vi "First Step.vi"(8 "error in (no error)":errorcluster, 11 "Varian Continuous.lvclass in":refnum<class "Varian Continuous.lvclass">) -> (0 "error out":errorcluster, 2 "Current Position":dbl, 3 "Varian Continuous.lvclass out":refnum<class "Varian Continuous.lvclass">)   [LabVIEW 2009, in "Varian Continuous.lvclass"]
doc: "(Dynamic) Reset the instrument and prepare to scan. Go to step #0 - the first step. If desired, the scanner may do this in a different way than usual (i.e. by preparing to move a long distance, or reset to home position.)"
uses:
  Varian Continuous.lvclass
  Instruments/Varian Magnet/Varian Magnet.lvclass
  Scanner/Scanner.lvclass
  Instruments/Varian Magnet/Varian Max Field.vi
  Varian Continuous.lvclass/Varian Continuous.ctl
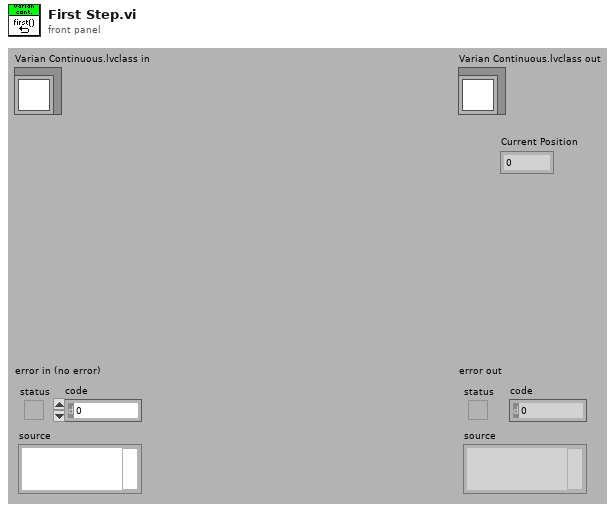
[diagram p1: front panel]
types:
  T1 = typedef "Scanner.lvclass/Range.ctl" = cluster{"xi":dbl, "xf":dbl, "dx":dbl, "Return to...?":bool, "Return to":dbl}
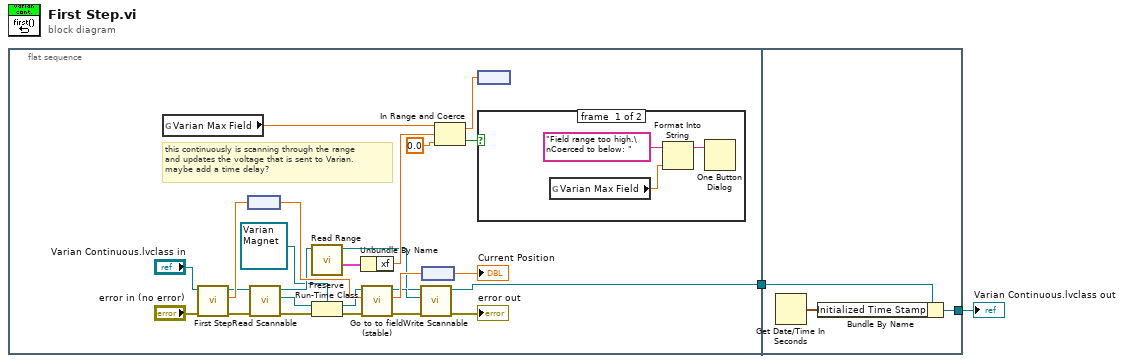
[diagram p0: block diagram]
diagram:
  n1 = flat-sequence {
    tunnel: [w10] -> w2
    tunnel: w2 -> [w32]
    tunnel: [w31] -> w1
    frame #0 {
      # "this continuously is scanning through the range\nand updates the voltage that is sent to Varian.\nmaybe add a time delay?"
      n2 = global read "Varian Max Field.vi" "Varian Max Field"() -> (w20:dbl[unit])
      n3 = call-parent "First Step.vi"("error in (no error)"="error in (no error)", "Scanner.lvclass in"="Varian Continuous.lvclass in") -> ("error out"=w13:errorcluster, "Current Position"=w25:dbl, "Scanner.lvclass out"=w21:refnum<class "Varian Continuous.lvclass">)  [unwired: 7 in]
      n4 = node(w25) -> (w24:dbl[unit])
      n5 = call-dynamic "Read Scannable.vi"("error in (no error)"=w13, "Scanner.lvclass in"=w21) -> ("error out"=w4:errorcluster, "Scannable.lvclass"=w7:refnum<class "Scannable.lvclass">, "Scanner.lvclass out"=w16:refnum<class "Varian Continuous.lvclass">)  [unwired: 7 in]
      n6 = call-dynamic "Read Range.vi"("Scanner.lvclass in"=w16) -> ("Range"=w15:T1, "Scanner.lvclass out"=w11:refnum<class "Varian Continuous.lvclass">)  [unwired: 5 in, 4 out]
      n7 = Preserve Run-Time Class(object in=w7, error in=w4, 2:refnum<class "Varian Magnet.lvclass"> refnum ("Varian Magnet.lvclass")) -> (object out=w5:refnum<class "Varian Magnet.lvclass">, error out=w3:errorcluster)
      n8 = Unbundle By Name(w15) -> ("xf"=w14:dbl)
      n9 = call "Go to to field (stable).vi"("error in"=w3, "Desired field"=w24, "varian in"=w5) -> ("error out"=w8:errorcluster, "Current field"=w22:dbl[unit], "varian out"=w12:refnum<class "Varian Magnet.lvclass">)  [unwired: 5 in, 1 out]
      n10 = call-dynamic "Write Scannable.vi"("error in (no error)"=w8, "Scannable.lvclass"=w12, "Scanner.lvclass in"=w11) -> ("error out"=→"error out":errorcluster, "Scanner.lvclass out"=w10:refnum<class "Varian Continuous.lvclass">)  [unwired: 7 out]
      n11 = node(w22) -> (→"Current Position":dbl)
      n12 = In Range and Coerce(upper limit=w20, x=w14, lower limit=dbl[unit] 0.0) -> (coerced(x)=w18:dbl[unit], In Range?=w17:bool)
      n13 = node(w18) -> ()  [unwired: 1 out]
      n14 = case shown="False" w17 {
        frame #0 {
          n15 = global read "Varian Max Field.vi" "Varian Max Field"() -> (w28:dbl[unit])
          n16 = Format Into String(initial string="Field range too high.\nCoerced to below: " ("message"), w28) -> (resulting string=w30:string)  [unwired: 2 in, 1 out]
          n17 = One Button Dialog(message=w30) -> ()  [unwired: 1 in, 1 out]
        }
        frame #1 {
        }
      }
    }
    frame #1 {
      n18 = Get Date/Time In Seconds() -> (seconds since 1Jan1904=w33:timestamp)
      n19 = Bundle By Name(cluster=w32, "Initialized Time Stamp"=w33) -> (w31:refnum<class "Varian Continuous.lvclass">)
    }
  }
  "Varian Continuous.lvclass out" <- w1
